vi "TestSuite_Init.vi"(7 "GUID (\"\")":string, 8 "error in (no error)":errorcluster, 9 "testSuiteStatusChanged EventRef":refnum<user-event>, 10 "tests (none)":refnum<class>[](array[class]), 11 "TestSuite in":refnum<class "TestSuite.lvclass">) -> (0 "error out":errorcluster, 3 "TestSuite out":refnum<class "TestSuite.lvclass">)   [LabVIEW 2013, in "TestSuite.lvclass"]
doc: "Initialize a TestSuite object with 'tests'. Tests are TestCase and/or TestSuite objects that have been initialized.\n\nThis method should be called inside of any instance of TestSuite.New method after the TestSuite test objects are created."
uses:
  TestSuite.lvclass
  suiteStatusChanged--Cluster.ctl
  suiteStatus--enum.ctl
  TestSuite.lvclass/TestSuite.ctl
  Libraries/VITesterUtilities.lvlib
panel:
  # "JKI VI Tester for LabVIEW\nhttp://jkisoft.com/vi-tester\nCopyright (C) 2007-2009, JKI <info@jkisoft.com>\nALL RIGHTS RESERVED"
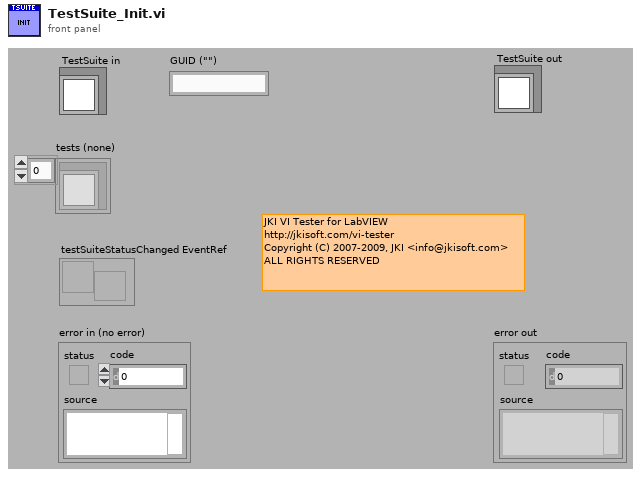
[diagram p1: front panel]
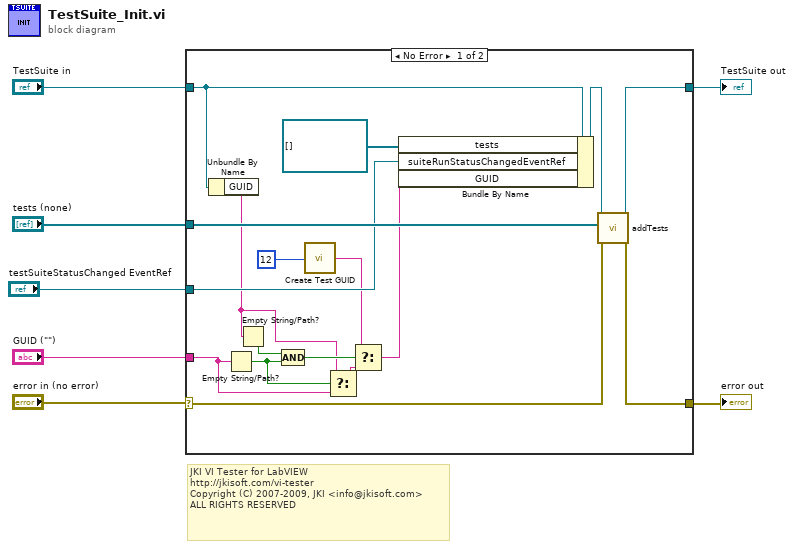
[diagram p0: block diagram]
diagram:
  # "JKI VI Tester for LabVIEW\nhttp://jkisoft.com/vi-tester\nCopyright (C) 2007-2009, JKI <info@jkisoft.com>\nALL RIGHTS RESERVED"
  n1 = case shown="No Error" "error in (no error)" {
    selector: "error in (no error)" -> [w18 w25]
    tunnel: "TestSuite in" -> [w15 w26]
    tunnel: [w22 w26] -> w6
    tunnel: [w21 w25] -> w4
    tunnel: "tests (none)" -> [w20 _]
    tunnel: "testSuiteStatusChanged EventRef" -> [w19 _]
    tunnel: "GUID (\"\")" -> [w10 _]
    frame No Error {
      n2 = Unbundle By Name(w15) -> ("GUID"=w11:string)
      n3 = Empty String/Path?(string/path=w10) -> (empty?=w12:bool)
      n4 = Empty String/Path?(string/path=w11) -> (empty?=w13:bool)
      n5 = Compound Arithmetic op=AND(w13, w12) -> (w14:bool)
      n6 = call "Create Test GUID.vi"("length"=12) -> ("random data"=w8:string)  [unwired: 4 in]
      n7 = Select(t=w11, s=w12, f=w10) -> (s? t:f=w9:string)
      n8 = Select(t=w8, s=w14, f=w9) -> (s? t:f=w16:string)
      n9 = Bundle By Name(cluster=w15, "tests"=refnum<class>[] [], "suiteRunStatusChangedEventRef"=w19, "GUID"=w16) -> (w23:refnum<class "TestSuite.lvclass">)
      n10 = call-dynamic "addTests.vi"("error in (no error)"=w18, "tests"=w20, "TestSuite in"=w23) -> ("error out"=w21:errorcluster, "TestSuite out"=w22:refnum<class "TestSuite.lvclass">)  [unwired: 7 in]
    }
    frame Error {
    }
  }
  "TestSuite out" <- w6
  "error out" <- w4
